vi "Read Settings.vi"(8 "error in (no error)":errorcluster, 11 "SRS850 in":refnum<class "SRS850.lvclass">) -> (0 "error out":errorcluster, 2 "Settings":string, 3 "SRS850 out":refnum<class "SRS850.lvclass">)   [LabVIEW 2015, in "SRS850.lvclass"]
uses:
  SRS850.lvclass
  Instrument/Instrument.lvclass
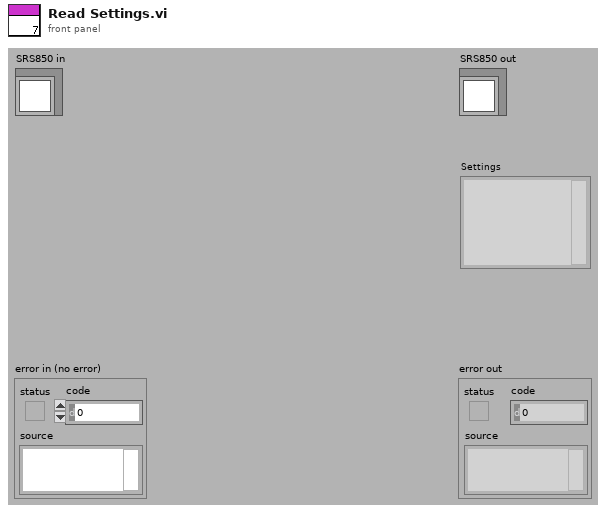
[diagram p1: front panel]
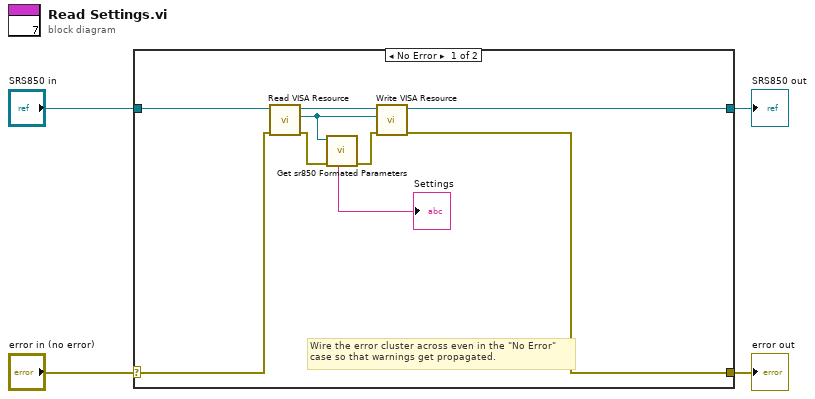
[diagram p0: block diagram]
diagram:
  n1 = case shown="No Error" "error in (no error)" {
    selector: "error in (no error)" -> [w10 w15]
    tunnel: [w7 w15] -> w3
    tunnel: [w11 w14] -> w1
    tunnel: "SRS850 in" -> [w12 w14]
    frame No Error {
      # "Wire the error cluster across even in the \"No Error\"\ncase so that warnings get propagated."
      n2 = call "Read VISA Resource.vi"("error in (no error)"=w10, "Instrument.lvclass in"=w12) -> ("error out"=w9:errorcluster, "VISA Resource"=w6:refnum<visa-resource-name>, "Instrument.lvclass out"=w13:refnum<class "SRS850.lvclass">)  [unwired: 7 out]
      n3 = call "Get sr850 Formated Parameters.VI"("error in (no error)"=w9, "VISA Resource Name"=w6) -> ("error out"=w8:errorcluster, "Parameters"=→"Settings":string)  [unwired: 1 in, 7 out]
      n4 = call "Write VISA Resource.vi"("error in (no error)"=w8, "VISA Resource"=w6, "Instrument.lvclass in"=w13) -> ("error out"=w7:errorcluster, "Instrument.lvclass out"=w11:refnum<class "SRS850.lvclass">)  [unwired: 7 out]
    }
    frame Error {
    }
  }
  "error out" <- w3
  "SRS850 out" <- w1
